vi "SubPanel_Oscilloscope_Block_Rev11.vi"(2 "error input":errorcluster, 3 "Oscilloscope Configuration Input Array":T2(array[cluster]) {"vertical coupling" items=["AC", "DC", "Ground"]}) -> (0 "error out":errorcluster, 1 "Oscilloscope Configuration Output Array":T2(array[cluster]) {"vertical coupling" items=["AC", "DC", "Ground"]})   [LabVIEW 2019]
uses:
  Controls/OscilloscopeBlockControl.ctl
  <instrlib>/niScope/Controls/niScope vertical coupling.ctl
  <instrlib>/niScope/Configure/Trigger/niScope Configure Trigger Software.vi
panel:
  out "Oscilloscope Configuration Array Indicator":T2(array[cluster]) {"vertical coupling" items=["AC", "DC", "Ground"]}
  in  "Remove An Oscilloscope":bool
  out "Horizontal:Actual Record Length":i32
  out "Configuration Errors":errorcluster
  in  "Oscilloscope Block Parameters":T3={"Oscilloscope"="", "channel names list"="", "vertical range"=10.0, "vertical coupling"=1, "Channel 0 50 ohms?"=FALSE, "50 ohm vertical range (V)"=10.0, "min record length"=1000, "min sample rate"=20000000.0} {"min sample rate" format="%^.2e"; "vertical coupling" items=["AC", "DC", "Ground"]}
  in  "EXIT SubVI":bool
  in  "Apply Configuration":bool
  # "Instructions\n\nSelect Oscilloscope Resource under \"Oscilloscope\"\n\nin a comma separate form (line 1, line 2, ...) type in the channel names of the device. \nIMPORTANT NOTE: \"line 1, line 2, ...\" will correspond to \"channel 0, channel 1, ...\" for each oscilloscope resource\n\nset the vertical range (no greater than 30)\n\nset the vertical coupling (dc) \n\nSet the channel 0 to 50 ohm impedance if you have something that requires 50 ohms to measure\n\nset 50 ohm vertical range if you have selected channel 0 50 ohms as true (ensure that it is no greater than 10\n\nmin record length (1000)\n\nmin sample rate (20e6) if you want a higher resolution, you increase the sample rate\n\npress apply configuration \n\nreview the instrument array above echoing your parameters created\n\nif you wish to remove a resource, select the oscilloscope resource in the \"oscillscope\" drop down\n\npress \"remove an oscilloscope\"\n\nonce fully configured, press \"EXIT\""
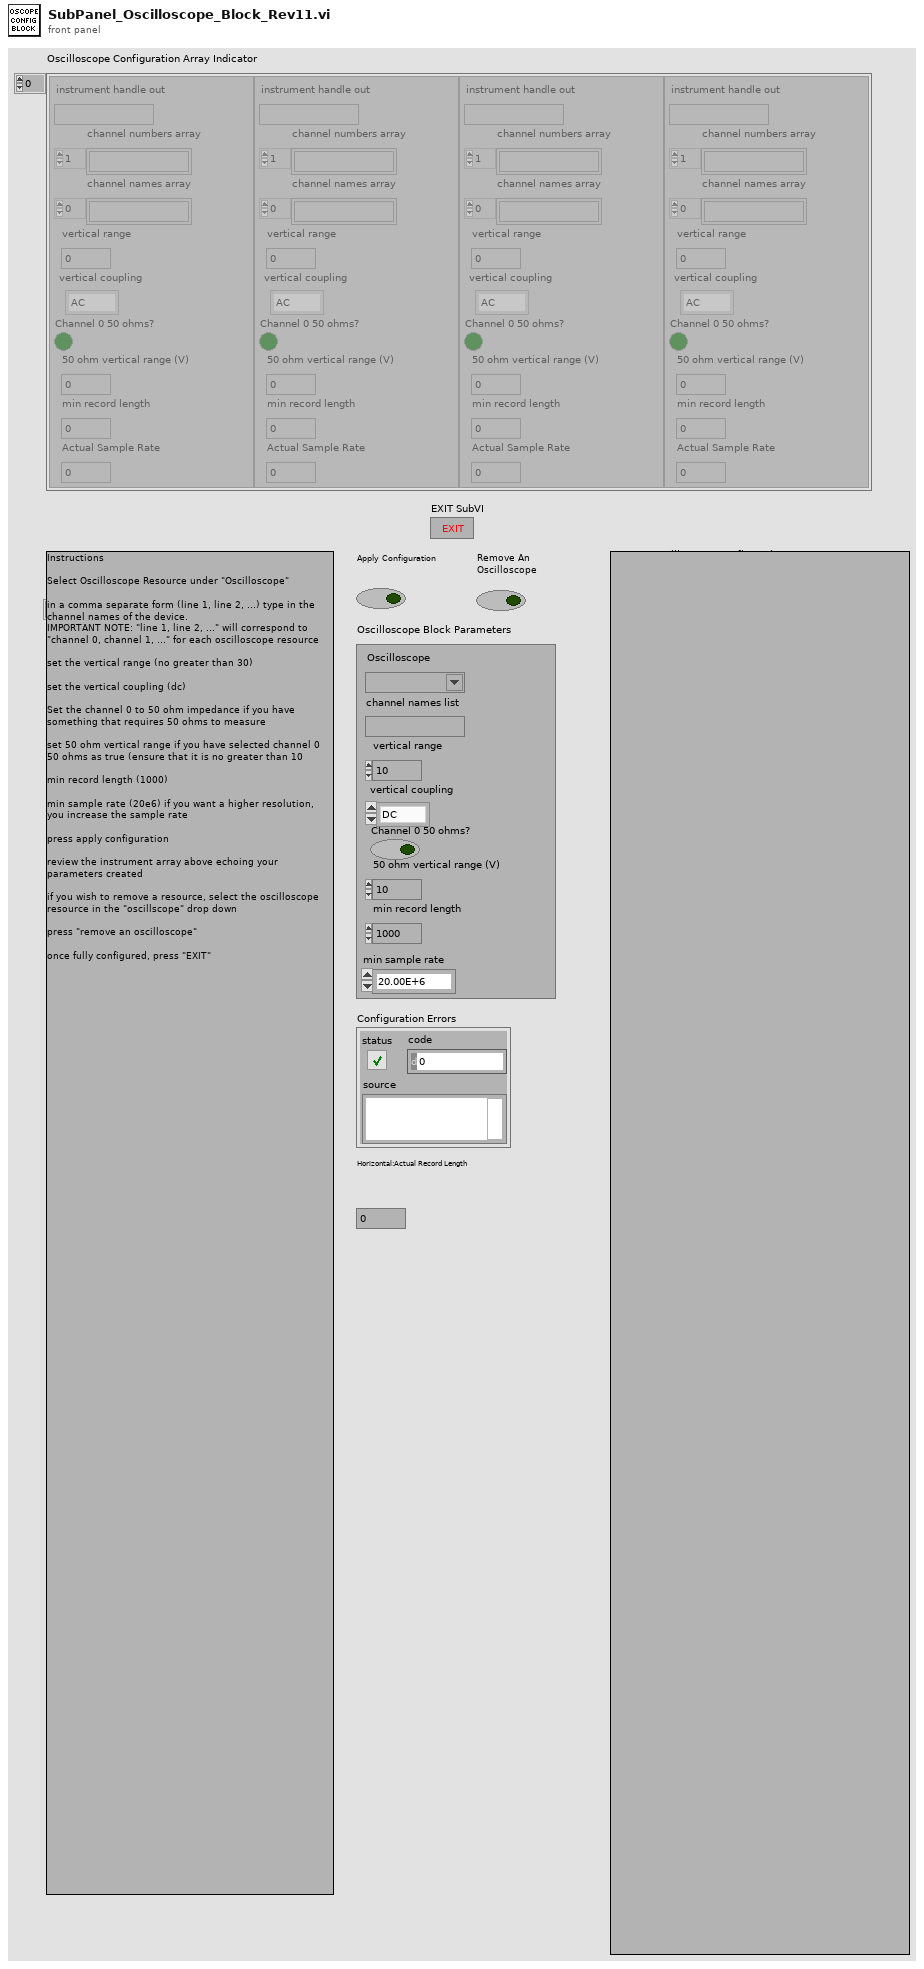
[diagram p1: front panel]
types:
  T1 = typedef "niScope vertical coupling.ctl" = i32
  T2 = cluster{"instrument handle out":refnum<k15>, "channel numbers array":string[], "channel names array":string[], "vertical range":dbl, "vertical coupling":T1, "Channel 0 50 ohms?":bool, "50 ohm vertical range (V)":dbl, "min record length":i32, "Actual Sample Rate":dbl}[]
  T3 = typedef "OscilloscopeBlockControl.ctl" = cluster{"Oscilloscope":refnum<k15>, "channel names list":string, "vertical range":dbl, "vertical coupling":T1, "Channel 0 50 ohms?":bool, "50 ohm vertical range (V)":dbl, "min record length":i32, "min sample rate":dbl}
  T4 = cluster{"instrument handle out":refnum<k15>, string[], string[], "vertical range":dbl, "vertical coupling":T1, "Channel 0 50 ohms?":bool, "50 ohm vertical range (V)":dbl, "min record length":i32, "Actual Sample Rate":dbl}
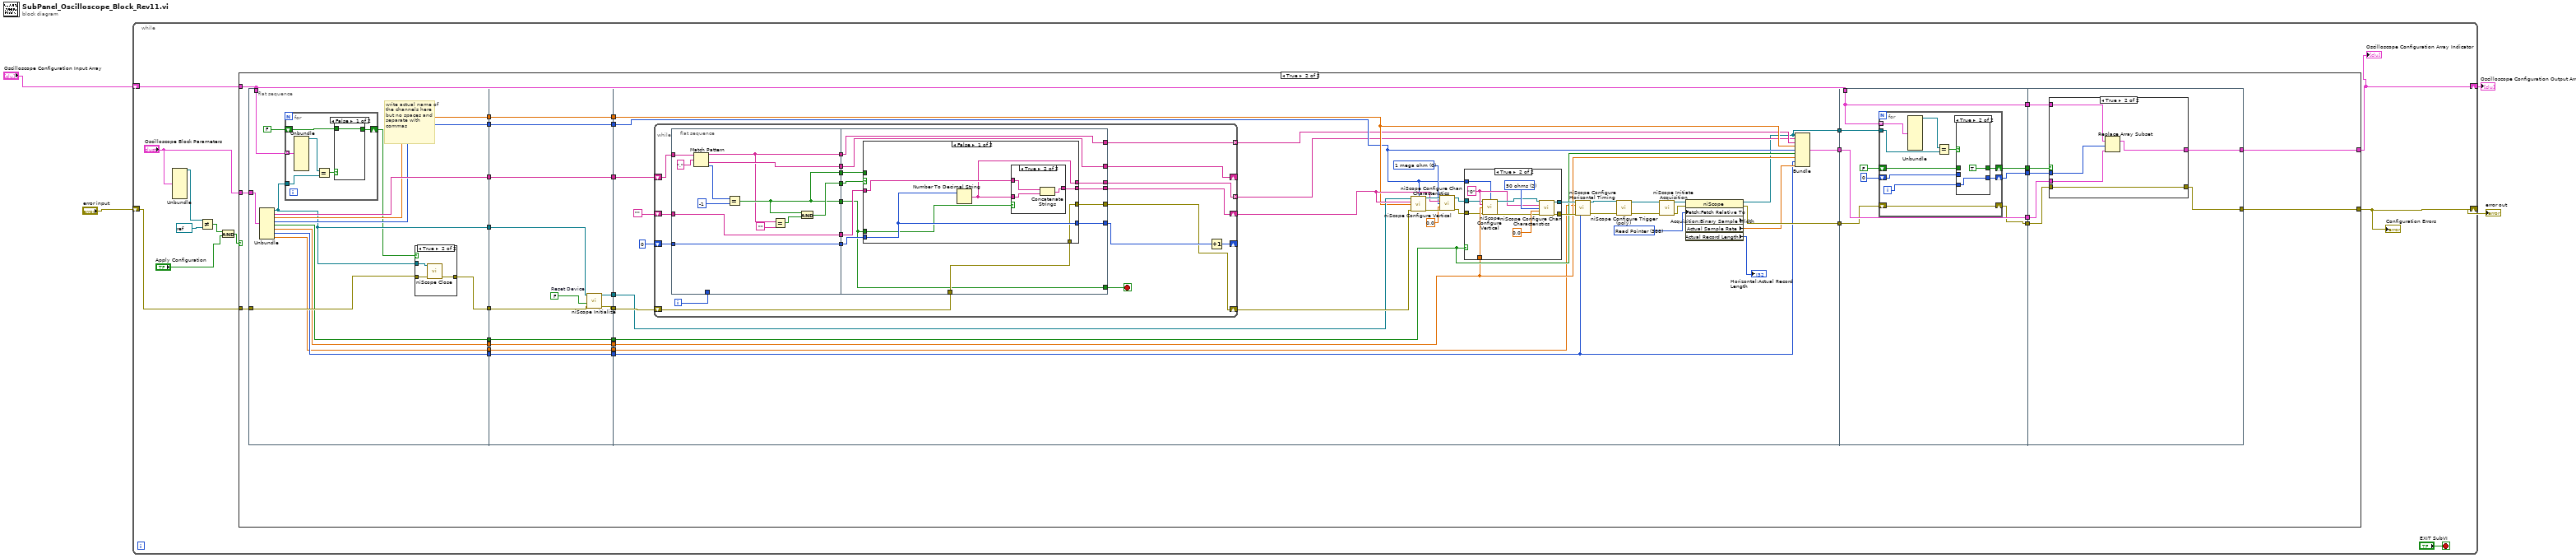
[diagram p0: block diagram]
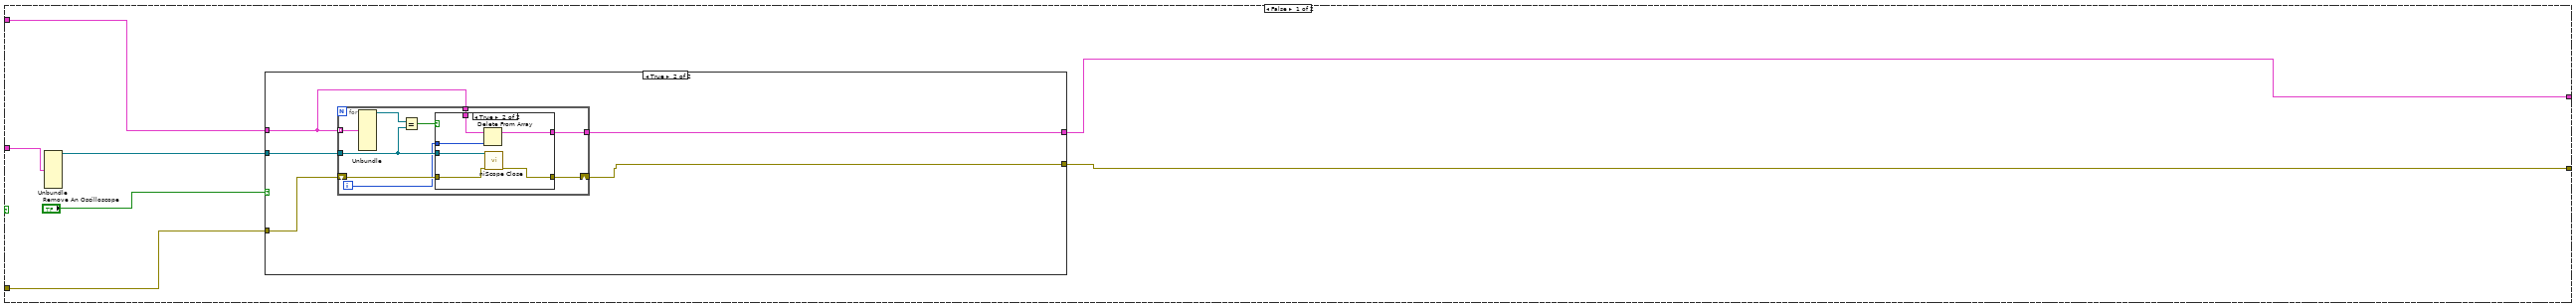
[diagram p2: hidden frame]
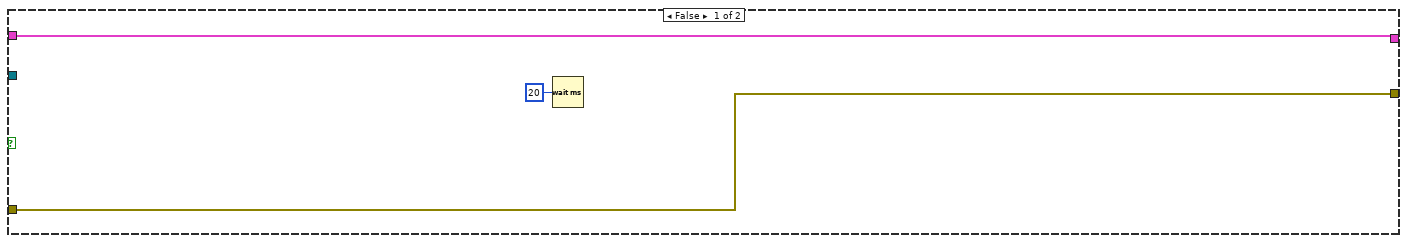
[diagram p3: hidden frame]
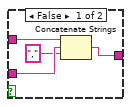
[diagram p7: hidden frame]
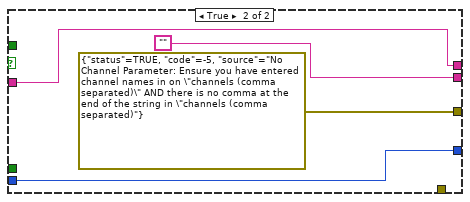
[diagram p8: hidden frame]
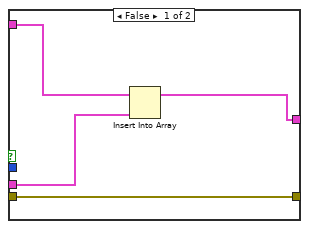
[diagram p11: hidden frame]
diagram:
  n1 = while {
    shift-right: [w15] -> w4
    shift-left: "error input" -> [w13]
    shift-right: [w5] -> w1
    shift-left: "Oscilloscope Configuration Input Array" -> [w12]
    stop <- "EXIT SubVI" stop-if-true
    n2 = Unbundle("Oscilloscope Block Parameters") -> ("Oscilloscope"=w9:refnum<k15>)  [unwired: 7 out]
    n3 = Not Equal?(x=w9, y=refnum<k15> refnum ("resource name")) -> (x != y?=w8:bool)
    n4 = And(x=w8, y="Apply Configuration") -> (x .and. y?=w6:bool)
    n5 = case shown="True" w6 {
      tunnel: w13 -> [w19 w78]
      tunnel: [w18 w73] -> w15
      tunnel: [w16 w72] -> w5
      tunnel: w12 -> [w17 w48]
      tunnel: "Oscilloscope Block Parameters" -> [w22 w49]
      frame False {
        n6 = Unbundle(w22) -> ("Oscilloscope"=w20:refnum<k15>)  [unwired: 7 out]
        n7 = case shown="True" "Remove An Oscilloscope" {
          tunnel: w20 -> [_ w30]
          tunnel: w19 -> [w25 w29]
          tunnel: [w25 w26] -> w18
          tunnel: w17 -> [w23 w28]
          tunnel: [w23 w27] -> w16
          frame False {
            n8 = Wait (ms)(milliseconds to wait=u32 20) -> ()  [unwired: 1 out]
          }
          frame True {
            n9 = for {
              tunnel: w28 -> [w39] mode=indexing
              tunnel: w30 -> [w36]
              shift-right: [w34] -> w26
              shift-left: w29 -> [w35]
              tunnel: w28 -> [w33]
              tunnel: [w31] -> w27
              i -> [w32]
              n10 = Unbundle(w39) -> ("instrument handle out"=w38:refnum<k15>)  [unwired: 8 out]
              n11 = Equal?(x=w38, y=w36) -> (x = y?=w37:bool)
              n12 = case shown="True" w37 {
                tunnel: w36 -> [_ w47]
                tunnel: w35 -> [w41 w46]
                tunnel: [w41 w45] -> w34
                tunnel: w33 -> [w40 w44]
                tunnel: w32 -> [_ w43]
                tunnel: [w40 w42] -> w31
                frame False {
                }
                frame True {
                  n13 = Delete From Array(array=w44, index=w43) -> (array with subset deleted=w42:T2)  [unwired: 1 in, 1 out]
                  n14 = call <instrlib>:"niScope Close.vi"("instrument handle"=w47, "error in"=w46) -> ("error out"=w45:errorcluster)  [unwired: 13 in]
                }
              }
            }
          }
        }
      }
      frame True {
        n15 = flat-sequence {
          tunnel: w78 -> [w92]
          tunnel: [w91] -> w74
          tunnel: [w81] -> w71
          tunnel: [w90] -> w70
          tunnel: [w89] -> w68
          tunnel: [w88] -> w66
          tunnel: [w87] -> w64
          tunnel: [w86] -> w62
          tunnel: [w85] -> w60
          tunnel: [w84] -> w58
          tunnel: w49 -> [w83]
          tunnel: w48 -> [w82]
          tunnel: [w112] -> w77
          tunnel: [w114] -> w76
          tunnel: [w113] -> w75
          tunnel: w74 -> [w115]
          tunnel: w71 -> [w111]
          tunnel: w70 -> [w112]
          tunnel: [w110] -> w69
          tunnel: w68 -> [w110]
          tunnel: [w109] -> w67
          tunnel: w66 -> [w109]
          tunnel: [w108] -> w65
          tunnel: w64 -> [w108]
          tunnel: [w107] -> w63
          tunnel: w62 -> [w107]
          tunnel: [w106] -> w61
          tunnel: w60 -> [w106]
          tunnel: [w105] -> w59
          tunnel: w58 -> [w105]
          tunnel: w75 -> [w127]
          tunnel: w76 -> [w130]
          tunnel: w77 -> [w131]
          tunnel: w69 -> [w126]
          tunnel: w67 -> [w125]
          tunnel: w65 -> [w124]
          tunnel: w63 -> [w123]
          tunnel: w61 -> [w122]
          tunnel: w59 -> [w121]
          tunnel: [w134] -> w57
          tunnel: [w128] -> w56
          tunnel: [w117] -> w55
          tunnel: w57 -> [w227]
          tunnel: w56 -> [w234]
          tunnel: w55 -> [w233]
          tunnel: w48 -> [w229]
          tunnel: [w226] -> w54
          tunnel: [w234] -> w53
          tunnel: [w230] -> w52
          tunnel: [w229] -> w51
          tunnel: [w228] -> w50
          tunnel: [w252] -> w72
          tunnel: [w249] -> w73
          tunnel: w54 -> [w250]
          tunnel: w53 -> [w251]
          tunnel: w52 -> [w255]
          tunnel: w51 -> [w254]
          tunnel: w50 -> [w253]
          frame #0 {
            # "write actual name of the channels here but no spaces and separate with commas"
            n16 = Unbundle(w83) -> ("Oscilloscope"=w81:refnum<k15>, "channel names list"=w90:string, "vertical range"=w89:dbl, "vertical coupling"=w88:T1, "Channel 0 50 ohms?"=w87:bool, "50 ohm vertical range (V)"=w86:dbl, "min record length"=w85:i32, "min sample rate"=w84:dbl)
            n17 = for {
              tunnel: w82 -> [w98] mode=indexing
              tunnel: w81 -> [w97]
              shift-right: [w94] -> w79
              shift-left: FALSE -> [w93]
              n18 = Unbundle(w98) -> ("instrument handle out"=w96:refnum<k15>)  [unwired: 8 out]
              n19 = Equal?(x=w96, y=w97) -> (x = y?=w95:bool)
              n20 = case shown="False" w95 {
                selector: w95 -> [_ w100]
                tunnel: [w99 w100] -> w94
                tunnel: w93 -> [w99 _]
                frame False {
                }
                frame True {
                }
              }
            }
            n21 = case shown="True" w79 {
              tunnel: w81 -> [_ w102]
              tunnel: w92 -> [w101 w104]
              tunnel: [w101 w103] -> w91
              frame False {
              }
              frame True {
                n22 = call <instrlib>:"niScope Close.vi"("instrument handle"=w102, "error in"=w104) -> ("error out"=w103:errorcluster)  [unwired: 13 in]
              }
            }
          }
          frame #1 {
            w116 = FALSE  # Reset Device
            n23 = call <instrlib>:"niScope Initialize.vi"("resource name"=w111, "reset device"=w116, "error in"=w115) -> ("instrument handle"=w113:refnum<k15>, "error out"=w114:errorcluster)  [unwired: 11 in]
          }
          frame #2 {
            w137 = 388 items=["Start"=482, "Trigger"=483, "Pretrigger"=477, "Now"=481, "Read Pointer"=388] ("Fetch:Fetch Relative To")
            w147 = u32 0 items=["1 mega ohm"=0, "50 ohms"=2] ("input impedance")
            n24 = while {
              shift-right: [w170] -> _
              shift-left: w131 -> [w171]
              shift-right: [w158] -> _
              shift-left: 0 -> [w163]
              shift-right: [w155] -> w148
              shift-left: "" -> [w161]
              tunnel: [w154] -> w120 mode=indexing
              shift-right: [w156] -> w151
              shift-left: w130 -> [w160]
              tunnel: [w152] -> w119 mode=indexing
              i -> [w169]
              stop <- w168 stop-if-true
              n25 = flat-sequence {
                tunnel: w171 -> [w181]
                tunnel: w169 -> [_]
                tunnel: [w179] -> w167
                tunnel: [w173] -> w166
                tunnel: [w174] -> w165
                tunnel: [w178] -> w164
                tunnel: w163 -> [w178]
                tunnel: [w177] -> w162
                tunnel: w161 -> [w177]
                tunnel: [w173] -> w157
                tunnel: [w172] -> w153
                tunnel: w167 -> [w195]
                tunnel: w166 -> [w186]
                tunnel: w165 -> [w194]
                tunnel: w164 -> [w192]
                tunnel: w162 -> [w191]
                tunnel: w160 -> [w190]
                tunnel: [w195] -> w170
                tunnel: [w186] -> w168
                tunnel: [w193] -> w155
                tunnel: [w189] -> w156
                tunnel: [w188] -> w159
                tunnel: w157 -> [w187]
                tunnel: [w185] -> w154
                tunnel: w153 -> [w185]
                tunnel: [w184] -> w152
                frame #0 {
                  n26 = Match Pattern(string=w181, regular expression=",") -> (before substring=w172:string, after substring=w179:string, offset past match=w183:i32)  [unwired: 1 in, 1 out]
                  n27 = Equal?(x=w183, y=-1) -> (x = y?=w173:bool)
                  n28 = Equal?(x=w172, y="") -> (x = y?=w175:bool)
                  n29 = And(x=w173, y=w175) -> (x .and. y?=w174:bool)
                }
                frame #1 {
                  n30 = case shown="False" w194 {
                    tunnel: [w197 ""] -> w193
                    tunnel: w192 -> [w201 w211]
                    tunnel: w191 -> [w199 w209]
                    tunnel: [w201 w211] -> w188
                    tunnel: w190 -> [w200 _]
                    tunnel: [w200 errorcluster {"status"=TRUE, "code"=-5, "source"="No Channel Parameter: Ensure you have entered channel names in on \"channels (comma separated)\" AND there is no comma at the end of the string in \"channels (comma separated)"} ("error out")] -> w189
                    tunnel: w187 -> [_ _]
                    tunnel: w186 -> [w198 _]
                    tunnel: [w196 w209] -> w184
                    frame False {
                      n31 = Number To Decimal String(number=w201) -> (decimal integer string=w196:string)  [unwired: 1 in]
                      n32 = case shown="True" w198 {
                        tunnel: w199 -> [w205 w208]
                        tunnel: w196 -> [w204 w207]
                        tunnel: [w202 w206] -> w197
                        frame False {
                          n33 = Concatenate Strings(w205, w204, "," ("string")) -> (w202:string)
                        }
                        frame True {
                          n34 = Concatenate Strings(w208, w207) -> (w206:string)
                        }
                      }
                    }
                    frame True {
                    }
                  }
                }
              }
              n35 = Increment(x=w159) -> (x+1=w158:i32)
            }
            n36 = call <instrlib>:"niScope Configure Vertical.vi"("instrument handle"=w127, "vertical coupling"=w125, "channels"=w148, "vertical range"=w126, "error in"=w151) -> ("instrument handle out"=w150:refnum<k15>, "error out"=w149:errorcluster)  [unwired: 9 in]
            n37 = call <instrlib>:"niScope Configure Chan Characteristics.vi"("instrument handle"=w150, "channels"=w148, "input impedance"=w147, "maximum input frequency"=0.0, "error in"=w149) -> ("instrument handle out"=w145:refnum<k15>, "error out"=w144:errorcluster)  [unwired: 9 in]
            n38 = case shown="True" w124 {
              tunnel: [w214 w225] -> w136
              tunnel: [w213 w224] -> w135
              tunnel: w123 -> [_ w218]
              tunnel: w145 -> [w214 w217]
              tunnel: w144 -> [w213 w216]
              tunnel: w125 -> [_ w215]
              frame False {
              }
              frame True {
                w222 = u32 2 items=["1 mega ohm"=0, "50 ohms"=2] ("input impedance")
                w219 = "0" ("channels")
                n39 = call <instrlib>:"niScope Configure Vertical.vi"("instrument handle"=w217, "vertical coupling"=w215, "channels"=w219, "vertical range"=w218, "error in"=w216) -> ("instrument handle out"=w221:refnum<k15>, "error out"=w220:errorcluster)  [unwired: 9 in]
                n40 = call <instrlib>:"niScope Configure Chan Characteristics.vi"("instrument handle"=w221, "channels"=w219, "input impedance"=w222, "maximum input frequency"=0.0, "error in"=w220) -> ("instrument handle out"=w225:refnum<k15>, "error out"=w224:errorcluster)  [unwired: 9 in]
              }
            }
            n41 = call <instrlib>:"niScope Configure Horizontal Timing.vi"("instrument handle"=w136, "min sample rate"=w121, "error in"=w135, "min record length"=w122) -> ("instrument handle out"=w143:refnum<k15>, "error out"=w142:errorcluster)  [unwired: 10 in]
            n42 = call-poly <instrlib>:"niScope Configure Trigger (poly).vi"("instrument handle"=w143, "error in"=w142) -> ("instrument handle out"=w140:refnum<k15>, "error out"=w141:errorcluster)  [unwired: 12 in]
            n43 = call <instrlib>:"niScope Initiate Acquisition.vi"("instrument handle"=w140, "error in"=w141) -> ("instrument handle out"=w139:refnum<k15>, "error out"=w138:errorcluster)  [unwired: 12 in]
            n44 = property class="niScope" props=["Fetch:Fetch Relative To", "Acquisition:Binary Sample Width", "Actual Sample Rate", "Actual Record Length"](reference=w139, error in=w138, "Fetch:Fetch Relative To"=w137) -> (reference out=w117:refnum<k15>, error out=w134:errorcluster, "Actual Sample Rate"=w129:dbl, "Actual Record Length"=→"Horizontal:Actual Record Length":i32)  [unwired: 1 out]
            n45 = Bundle("instrument handle out"=w117, w119, w120, "vertical range"=w126, "vertical coupling"=w125, "Channel 0 50 ohms?"=w124, "50 ohm vertical range (V)"=w123, "min record length"=w122, "Actual Sample Rate"=w129) -> (w128:T4)  [unwired: 1 in]
          }
          frame #3 {
            n46 = for {
              tunnel: w229 -> [w244] mode=indexing
              tunnel: w233 -> [w242]
              shift-right: [w239] -> w230
              shift-left: FALSE -> [w240]
              shift-right: [w237] -> w228
              shift-left: 0 -> [w238]
              shift-right: [w235] -> w226
              shift-left: w227 -> [w235]
              i -> [w236]
              n47 = Unbundle(w244) -> ("instrument handle out"=w243:refnum<k15>)  [unwired: 8 out]
              n48 = Equal?(x=w243, y=w242) -> (x = y?=w241:bool)
              n49 = case shown="True" w241 {
                tunnel: w240 -> [w246 _]
                tunnel: [w246 TRUE] -> w239
                tunnel: w238 -> [w245 _]
                tunnel: [w245 w247] -> w237
                tunnel: w236 -> [_ w247]
                frame False {
                }
                frame True {
                }
              }
            }
          }
          frame #4 {
            n50 = case shown="True" w255 {
              tunnel: w254 -> [w259 w264]
              tunnel: w251 -> [w258 w263]
              tunnel: w253 -> [_ w262]
              tunnel: [w257 w261] -> w252
              tunnel: [w256 w260] -> w249
              tunnel: w250 -> [w256 w260]
              frame False {
                n51 = Insert Into Array(array=w259, new element=w258) -> (w257:T2)  [unwired: 1 in]
              }
              frame True {
                n52 = Replace Array Subset(array=w264, new element=w263, index=w262) -> (w261:T2)
              }
            }
          }
        }
      }
    }
    "Configuration Errors" <- w15
    "Oscilloscope Configuration Array Indicator" <- w5
  }
  "error out" <- w4
  "Oscilloscope Configuration Output Array" <- w1
